vi "TF_StrainGauge2ForceV2.vi"(0 "Action (Read)":T2=enum."Read", 2 "Strain Gauge Value [V]":dbl, 3 "ETH Mike Model":T1) -> (5 "Force [N]":dbl)   [LabVIEW 2019]
uses:
  ReadOnlyGlobalActions.ctl
  ETHMikeModel.ctl
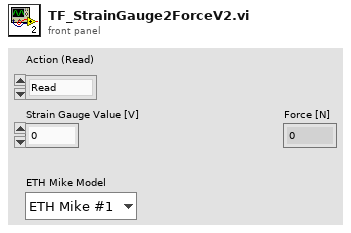
[diagram p1: front panel]
types:
  T1 = typedef "ETHMikeModel.ctl" = enum16{"ETH Mike #1", "ETH Mike #2", "ETH Mike #3", "ETH Mike #4", "ETH MIKE #5"}
  T2 = typedef "ReadOnlyGlobalActions.ctl" = enum16{"Initialize", "Read"}
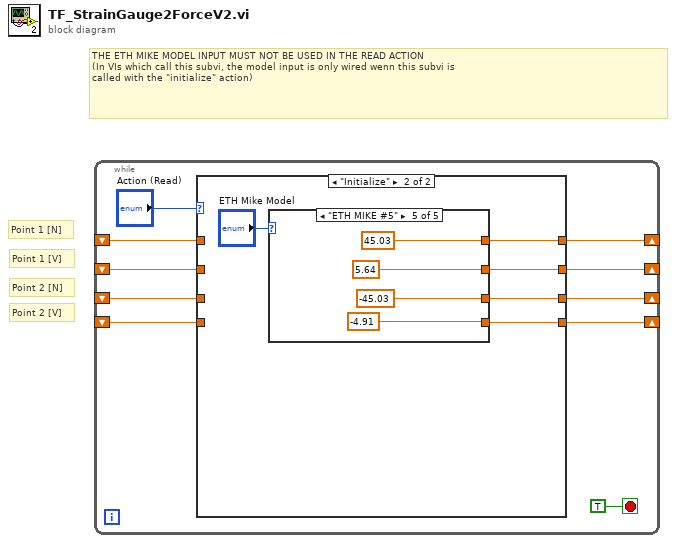
[diagram p0: block diagram]
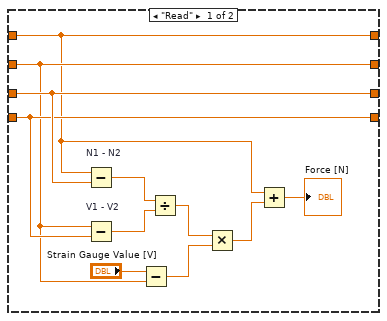
[diagram p2: hidden frame]
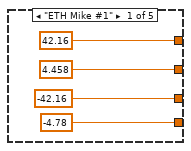
[diagram p3: hidden frame]
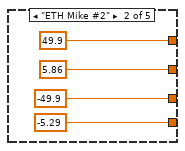
[diagram p4: hidden frame]
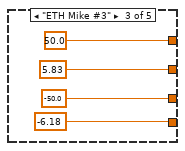
[diagram p5: hidden frame]
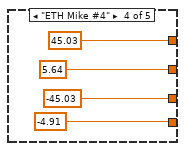
[diagram p6: hidden frame]
diagram:
  # "THE ETH MIKE MODEL INPUT MUST NOT BE USED IN THE READ ACTION\n(In VIs which call this subvi, the model input is only wired wenn this subvi is\ncalled with the \"initialize\" action)"
  # "Point 2 [V]"
  # "Point 2 [N]"
  # "Point 1 [V]"
  # "Point 1 [N]"
  n1 = while {
    shift-right: [w9] -> _
    shift-left: _ -> [w8]
    shift-right: [w6] -> _
    shift-left: _ -> [w5]
    shift-right: [w4] -> _
    shift-left: _ -> [w2]
    shift-right: [w3] -> _
    shift-left: _ -> [w1]
    stop <- TRUE stop-if-true
    n2 = case shown="\"Initialize\"" "Action (Read)" {
      tunnel: [w12 w25] -> w9
      tunnel: w8 -> [w12 _]
      tunnel: [w15 w24] -> w6
      tunnel: w5 -> [w15 _]
      tunnel: [w21 w23] -> w4
      tunnel: [w20 w22] -> w3
      tunnel: w2 -> [w21 _]
      tunnel: w1 -> [w20 _]
      frame "Read" {
        n3 = Subtract "N1 - N2"(x=w12, y=w21) -> (x-y=w19:dbl)
        n4 = Subtract "V1 - V2"(x=w15, y=w20) -> (x-y=w18:dbl)
        n5 = Subtract(x="Strain Gauge Value [V]", y=w15) -> (x-y=w14:dbl)
        n6 = Divide(x=w19, y=w18) -> (x/y=w17:dbl)
        n7 = Multiply(x=w17, y=w14) -> (x*y=w13:dbl)
        n8 = Add(x=w12, y=w13) -> (x+y=→"Force [N]":dbl)
      }
      frame "Initialize" {
        n9 = case shown="\"ETH MIKE #5\"" "ETH Mike Model" {
          tunnel: [42.16 ("Point 1 [N]") 49.9 ("Point 1 [N]") 50.0 45.03 45.03] -> w25
          tunnel: [4.458 ("Point 1 [V]") 5.86 ("Point 1 [V]") 5.83 5.64 5.64] -> w24
          tunnel: [-42.16 ("Point 2 [N]") -49.9 ("Point 2 [N]") -50.0 -45.03 -45.03] -> w23
          tunnel: [-4.78 ("Point 2 [V]") -5.29 ("Point 2 [V]") -6.18 -4.91 -4.91] -> w22
          frame "ETH Mike #1" {
          }
          frame "ETH Mike #2" {
          }
          frame "ETH Mike #3" {
          }
          frame "ETH Mike #4" {
          }
          frame "ETH MIKE #5" {
          }
        }
      }
    }
  }
